vi "Get Users Groups.vi"(8 "error in (no error)":errorcluster, 11 "userName":string) -> (0 "error out":errorcluster, 3 "groups":string[](array[string]))   [LabVIEW 2017, in "Windows Security.lvlib"]
doc: "Returns the user's groups."
uses:
  Windows Security.lvlib
  System.DirectoryServices.AccountManagement
panel:
  in  "domain?":bool=TRUE
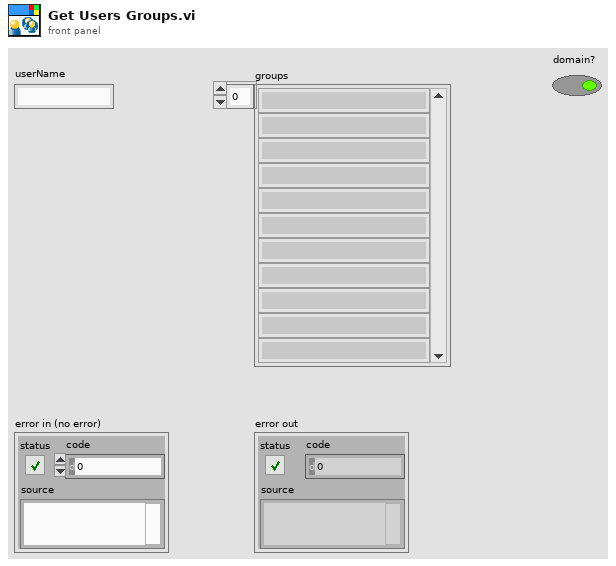
[diagram p1: front panel]
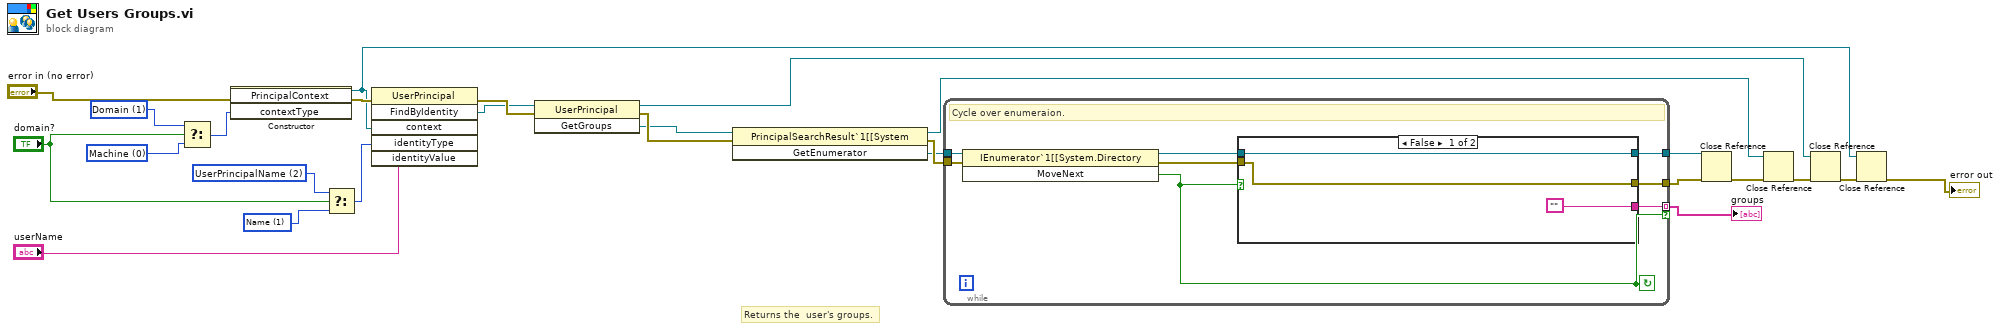
[diagram p0: block diagram]
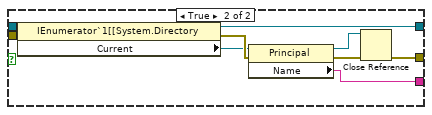
[diagram p2: hidden frame]
diagram:
  w4 = 1 items=["SamAccountName", "Name", "UserPrincipalName", "DistinguishedName", "Sid", "Guid"] ("identityType")
  w9 = 0 items=["Machine", "Domain", "ApplicationDirectory"] ("contextType")
  w10 = 1 items=["Machine", "Domain", "ApplicationDirectory"] ("contextType")
  w7 = 2 items=["SamAccountName", "Name", "UserPrincipalName", "DistinguishedName", "Sid", "Guid"] ("identityType")
  # "Returns the  user's groups."
  n1 = Select(t=w10, s="domain?", f=w9) -> (s? t:f=w8:i32)
  n2 = constructor class="PrincipalContext"(error in="error in (no error)", "contextType"=w8) -> (reference out=w1:refnum<k24>, error out=w11:errorcluster)  [unwired: 2 in, 2 out]
  n3 = Select(t=w7, s="domain?", f=w4) -> (s? t:f=w6:i32)
  n4 = invoke class="UserPrincipal" method="FindByIdentity"(error in=w11, "context"=w1, "identityType"=w6, "identityValue"="userName") -> (error out=w26:errorcluster, "FindByIdentity"=w13:refnum<k24>)  [unwired: 2 in, 4 out]
  n5 = invoke class="UserPrincipal" method="GetGroups"(reference=w13, error in=w26) -> (reference out=w15:refnum<k24>, error out=w24:errorcluster, "rvices.AccountManagement, Version=0.0.0.0, Culture=neutral, PublicKeyToken=b77a5c561934e089\tGetGroups"=w23:refnum<k24>)  [unwired: 1 in]
  n6 = invoke class="PrincipalSearchResult`1[[System" method="GetEnumerator"(reference=w23, error in=w24) -> (reference out=w16:refnum<k24>, error out=w25:errorcluster, "GetEnumerator"=w22:refnum<k24>)  [unwired: 1 in]
  n7 = while {
    tunnel: w22 -> [w34]
    tunnel: [w32] -> w21 mode=indexing if=w28
    tunnel: w25 -> [w31]
    tunnel: [w29] -> w20
    tunnel: [w27] -> w17
    stop <- w28 continue-if-true
    # "Cycle over enumeraion."
    n8 = invoke class="IEnumerator`1[[System.Directory" method="MoveNext"(reference=w34, error in=w31) -> (reference out=w33:refnum<k24>, error out=w30:errorcluster, "MoveNext"=w28:bool)  [unwired: 1 in]
    n9 = case shown="False" w28 {
      tunnel: w33 -> [w35 w44]
      tunnel: ["" w43] -> w32
      tunnel: w30 -> [w37 w42]
      tunnel: [w37 w39] -> w29
      tunnel: [w35 w38] -> w27
      frame False {
      }
      frame True {
        n10 = property class="IEnumerator`1[[System.Directory"(reference=w44, error in=w42) -> (reference out=w38:refnum<k24>, error out=w46:errorcluster, "Current"=w45:refnum<k24>)
        n11 = property class="Principal"(reference=w45, error in=w46) -> (reference out=w40:refnum<k24>, error out=w41:errorcluster, "Name"=w43:string)
        n12 = Close Reference(reference=w40, error in (no error)=w41) -> (error out=w39:errorcluster)
      }
    }
  }
  "groups" <- w21
  n13 = Close Reference(reference=w17, error in (no error)=w20) -> (error out=w18:errorcluster)
  n14 = Close Reference(reference=w16, error in (no error)=w18) -> (error out=w19:errorcluster)
  n15 = Close Reference(reference=w15, error in (no error)=w19) -> (error out=w3:errorcluster)
  n16 = Close Reference(reference=w1, error in (no error)=w3) -> (error out=→"error out":errorcluster)
